vi "Challenge-1.vi"   [LabVIEW 2014, in "Diaz_Razo_5th_LegoRobotics_11-29-16.lvrbt"]
uses:
  Diaz_Razo_5th_LegoRobotics_11-29-16.lvrbt
  <vilib>/NXT/Block Support/NXT_InputPort.ctl
  <vilib>/NXT/Block Support/NXT_OutputPort.ctl
  <vilib>/NXT/NXTIO Xnodes/NXTIONodeSubVIs/NXTMoveMotors.vi
  <vilib>/NXT/Dual Mode Library/Waits/Wait_Num.vi
  <vilib>/NXT/NXTIO Xnodes/NXTIONodeSubVIs/LEGOStopAllMotors.vi
  <vilib>/NXT/NXTIO Xnodes/AddressXNode/NXTIOAddress.xnode
  <vilib>/NXT/NXTIO Xnodes/NXTIOXNode/NXTIO.xnode
  <vilib>/NXT/Subs/LVHSConnector.ctl
  <vilib>/NXT/LegoClasses/BrickReference/BrickReference.lvclass
types:
  T1 = typedef "NXT_OutputPort.ctl" = u8
  T2 = typedef "NXT_InputPort.ctl" = u32
  T3 = typedef "LVHSConnector.ctl" = refnum<class "BrickReference.lvclass">
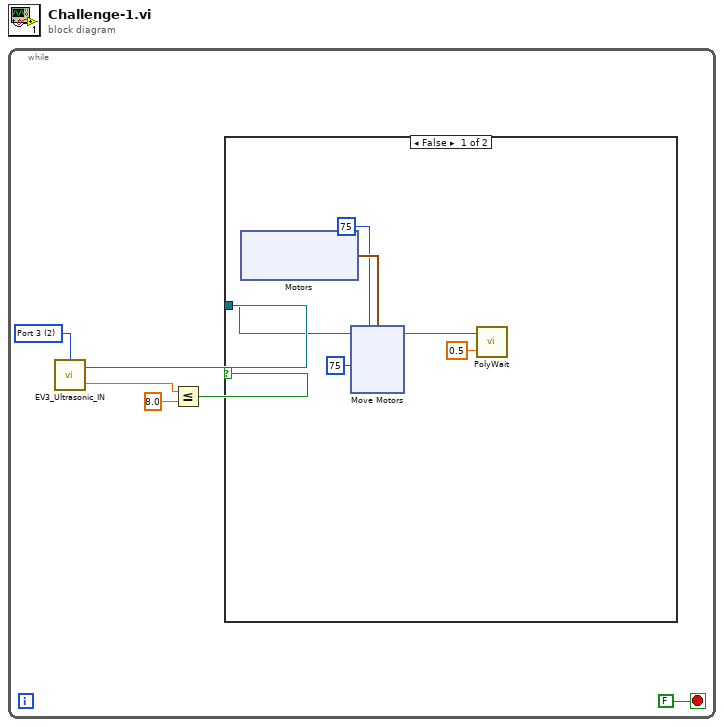
[diagram p0: block diagram]
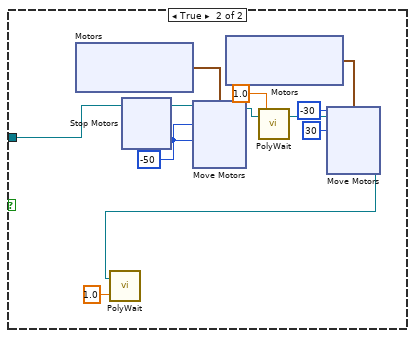
[diagram p2: hidden frame]
diagram:
  n1 = while {
    stop <- FALSE stop-if-true
    w5 = T2 2 items=["Port 1", "Port 2", "Port 3", "Port 4"] ("Port (Port 1)")
    n2 = call <vilib>:"EV3_Ultrasonic_IN.vi"("Port (Port 1)"=w5) -> ("Inches"=w4:sgl, "NXT/EV3"=w1:T3)  [unwired: 2 in]
    n3 = Less Or Equal?(x=w4, y=sgl 8.0) -> (x <= y?=w2:bool)
    n4 = case shown="False" w2 {
      tunnel: w1 -> [w7 w25]
      frame False {
        n5 = xnode "Motors"() -> ("Motor"=w12:cluster{"Port":T1, "Port":T1})
        n6 = xnode "Move Motors"("Power/Speed 2"=i8 75, "Power/Speed 1"=i8 75, "Motors"=w12, "NXT/EV3"=w7) -> ("NXT/EV3"=w9:T3)
        n7 = call-poly <vilib>:"PolyWait.vi"("Time (1 sec)"=sgl 0.5, "NXT/EV3"=w9) -> ()  [unwired: 2 in, 1 out]
      }
      frame True {
        w32 = i8 -50 ("Power/Speed 1")
        n8 = xnode "Motors"() -> ("Motor"=w33:cluster{"Port":T1, "Port":T1})
        n9 = xnode "Stop Motors"("NXT/EV3"=w25) -> ("NXT/EV3"=w24:T3)  [unwired: 1 in]
        n10 = xnode "Move Motors"("Power/Speed 2"=w32, "Power/Speed 1"=w32, "Motors"=w33, "NXT/EV3"=w24) -> ("NXT/EV3"=w31:T3)
        n11 = xnode "Motors"() -> ("Motor"=w28:cluster{"Port":T1, "Port":T1})
        n12 = call-poly <vilib>:"PolyWait.vi"("Time (1 sec)"=sgl 1.0, "NXT/EV3"=w31) -> ("NXT/EV3"=w29:T3)  [unwired: 2 in]
        n13 = xnode "Move Motors"("Power/Speed 2"=i8 -30, "Power/Speed 1"=i8 30, "Motors"=w28, "NXT/EV3"=w29) -> ("NXT/EV3"=w23:T3)
        n14 = call-poly <vilib>:"PolyWait.vi"("Time (1 sec)"=sgl 1.0, "NXT/EV3"=w23) -> ()  [unwired: 2 in, 1 out]
      }
    }
  }
